vi "Stop Core.vi"(10 "final error code":i32, 11 "File Actor in":refnum<class "File Actor.lvclass">) -> (3 "File Actor out":refnum<class "File Actor.lvclass">)   [LabVIEW 2016, in "File Library.lvlib" / "File Actor.lvclass"]
doc: "(<B>Filename</B>: Actor Framework.lvlib:Actor.lvclass:Stop Core.vi)\n\nDefines what the actor does before it stops. Use the <B>final error code</B> input to determine whether the actor shut down in response to an error.\n\nBy default, this method does nothing. A descendant class may override it to define behavior, such as shutting down any processes the actor initiated in its override of the Actor Core method."
uses:
  File Actor.lvclass
  C:/Program Files (x86)/National Instruments/LabVIEW 2016/vi.lib/MSR Consulting, LLC/General Reuse/SuperActor/SuperActor.lvclass
  File Actor.lvclass/File Actor.ctl
  <vilib>/MSR Consulting, LLC/General Reuse/SuperActor/SuperActor.lvclass/SuperActor.ctl
  <vilib>/MSR Consulting, LLC/General Reuse/SuperActor/Read ID.vi
  <vilib>/MSR Consulting, LLC/General Reuse/SuperActor/Read Log Session.vi
  <vilib>/MSR Consulting, LLC/General Reuse/Session APIs/_Session Fwk/Session - Root.lvclass
  <vilib>/MSR Consulting, LLC/General Reuse/SuperActor/SuperActor.lvclass
  <vilib>/MSR Consulting, LLC/General Reuse/Session APIs/Session Log/System Log.lvclass
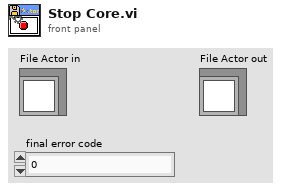
[diagram p1: front panel]
types:
  T1 = typedef "Session - Root.lvclass/Session Handle.ctl" = refnum<data-value>
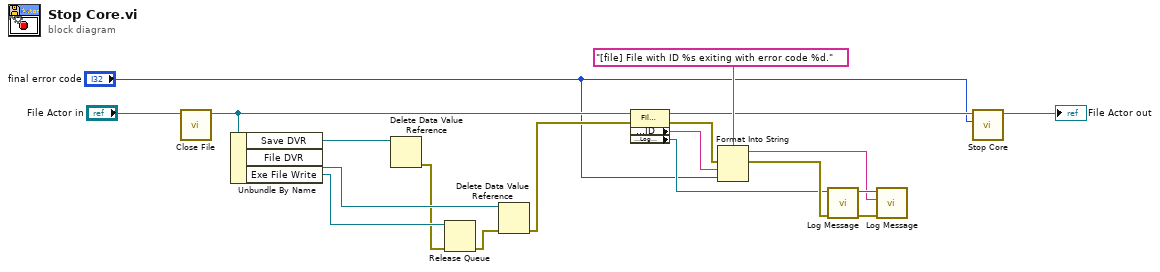
[diagram p0: block diagram]
diagram:
  n1 = call "Close File.vi"("File Actor in"="File Actor in") -> ("File Actor out"=w10:refnum<class "File Actor.lvclass">)  [unwired: 9 in, 1 out]
  n2 = Unbundle By Name(w10) -> ("Save DVR"=w17:refnum<data-value>, "File DVR"=w18:refnum<data-value>, "Exe File Write"=w16:refnum<queue>)
  n3 = Delete Data Value Reference(data value reference=w17) -> (error out=w13:errorcluster)  [unwired: 1 in, 1 out]
  n4 = Release Queue(queue=w16, error in (no error)=w13) -> (error out=w8:errorcluster)  [unwired: 1 in, 2 out]
  n5 = Delete Data Value Reference(data value reference=w18, error in=w8) -> (error out=w12:errorcluster)  [unwired: 1 out]
  n6 = property class="File Actor.lvclass"(reference=w10, error in=w12) -> (reference out=w4:refnum<class "File Actor.lvclass">, error out=w11:errorcluster, "Accessors:ID"=w14:string, "Accessors:Log Session"=w5:T1)
  n7 = Format Into String(format string="[file] File with ID %s exiting with error code %d.", error in=w11, w14, "final error code") -> (resulting string=w6:string, error out=w9:errorcluster)  [unwired: 1 in]
  n8 = call <vilib>:"Log Message.vi"("error in"=w9, "session in"=w5) -> ("error out"=w2:errorcluster, "session out"=w7:T1)  [unwired: 8 in]
  n9 = call <vilib>:"Log Message.vi"("error in"=w2, "MSG In"=w6, "session in"=w7) -> ()  [unwired: 7 in, 2 out]
  n10 = call-parent "Stop Core.vi"("final error code"="final error code", "Ex Nested in"=w4) -> ("Ex Nested out"=→"File Actor out":refnum<class "File Actor.lvclass">)  [unwired: 9 in]
